vi "Request Buffer from Server.vi"(8 "error in (no error)":errorcluster, 9 "timeout ms (25000)":i32=25000, 10 "buffer descriptor":T1={"buffer type"=enum."Engine", "plugin id"=-1, "group id"=-1, "transfer id"=-1, "offset"=0, "length"=-1}, 11 "server ID in":refnum<k5>) -> (0 "error out":errorcluster, 1 "timed out?":bool, 3 "server ID out":refnum<k5>)   [LabVIEW 2020, in "DSF Core.lvlib"]
uses:
  DSF Core.lvlib
  DSF Buffer Subset Descriptor.ctl
  Typedefs/DSF Buffer Type.ctl
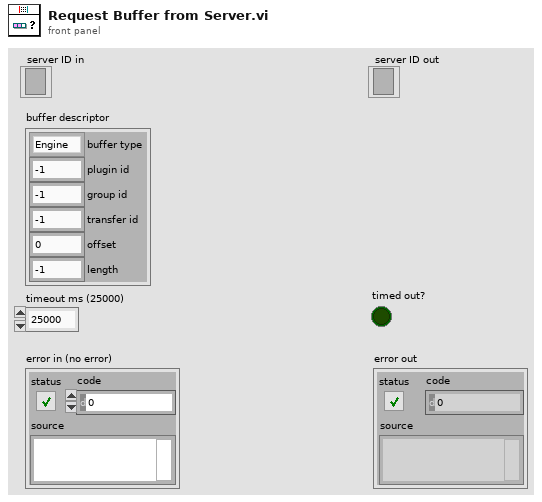
[diagram p1: front panel]
types:
  T1 = typedef "DSF Core.lvlib/DSF Buffer Subset Descriptor.ctl" = cluster{"buffer type":T2, "plugin id":i32, "group id":i32, "transfer id":i32, "offset":u64, "length":i64}
  T2 = typedef "DSF Core.lvlib/DSF Buffer Type.ctl" = enum16{"Engine", "String"}
  T3 = enum16{"big-endian, network order", "native, host order", "little-endian"}
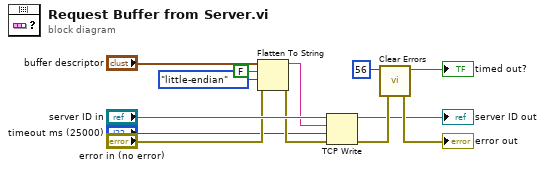
[diagram p0: block diagram]
diagram:
  n1 = Flatten To String(anything="buffer descriptor", prepend array or string size? (T)=FALSE, byte order (0:big-endian, network order)=T3."little-endian", error in (no error)="error in (no error)") -> (data string=w8:string, error out=w10:errorcluster)  [unwired: 1 out]
  n2 = TCP Write(connection ID="server ID in", data in=w8, error in (no error)=w10, 9:"timeout ms (25000)") -> (connection ID out=→"server ID out":refnum<k5>, error out=w7:errorcluster)  [unwired: 1 out]
  n3 = call <vilib>:"Clear Errors.vi"("error in (no error)"=w7, "specific error code to clear (0: all)"=56) -> ("error out"=→"error out":errorcluster, "specific error cleared?"=→"timed out?":bool)  [unwired: 4 in]
